vi "Voltage Display.vi"(0 "RedPitaya connection in":refnum<k5>, 2 "Vertical Offset":dbl=20.1 min=-20.0 max=20.1, 3 "Vertical Scale":dbl=-1.0, 5 "error in":errorcluster, 8 "Channel #":u16(ring)=1 items=["Channel 1"=1, "Channel 2"=2], 12 "timeout ms (2000)":i32=2000) -> (14 "RedPitaya connection out":refnum<k5>, 19 "error out":errorcluster)   [LabVIEW 2021, in "RedPitaya.lvlib"]
doc: "Sets vertical offset and scale of selected channel"
uses:
  RedPitaya.lvlib
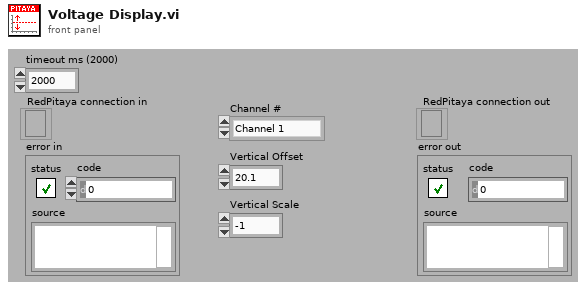
[diagram p1: front panel]
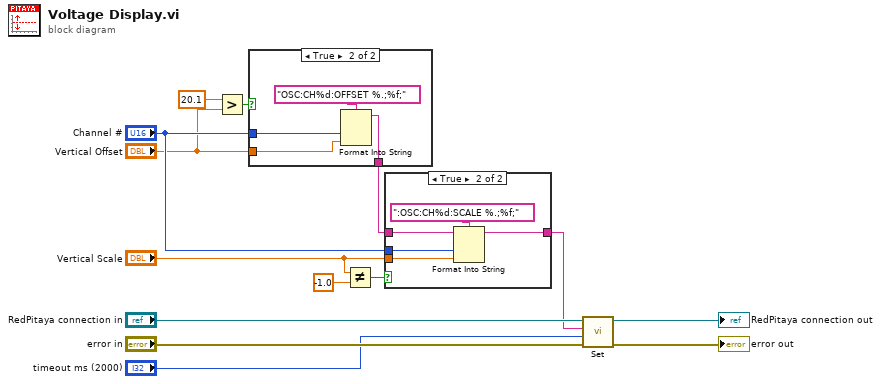
[diagram p0: block diagram]
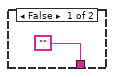
[diagram p3: hidden frame]
diagram:
  n1 = Greater?(x=20.1, y="Vertical Offset") -> (0:w7:bool)
  n2 = case shown="True" w7 {
    tunnel: "Vertical Offset" -> [_ w18]
    tunnel: ["" w17] -> w10
    tunnel: "Channel #" -> [_ w16]
    frame False {
    }
    frame True {
      n3 = Format Into String(format string="OSC:CH%d:OFFSET %.;%f;", w16, w18) -> (resulting string=w17:string)  [unwired: 2 in, 1 out]
    }
  }
  n4 = Not Equal?(x="Vertical Scale", y=-1.0) -> (x != y?=w4:bool)
  n5 = case shown="True" w4 {
    tunnel: w10 -> [w20 w25]
    tunnel: "Channel #" -> [_ w23]
    tunnel: "Vertical Scale" -> [_ w22]
    tunnel: [w20 w21] -> w8
    frame False {
    }
    frame True {
      n6 = Format Into String(format string=":OSC:CH%d:SCALE %.;%f;", initial string=w25, w23, w22) -> (resulting string=w21:string)  [unwired: 1 in, 1 out]
    }
  }
  n7 = call "Set.vi"("error in"="error in", "timeout ms (2000)"="timeout ms (2000)", "SCPI Message"=w8, "RedPitaya connection in"="RedPitaya connection in") -> ("error out"=→"error out":errorcluster, "RedPitaya connection out"=→"RedPitaya connection out":refnum<k5>)  [unwired: 5 in, 1 out]
